vi "GetVideoInOptionsConfig.vi"(7 "HTTP_address":string, 8 "error in (no error)":errorcluster, 10 "Value":T2, 11 "Refnum in":T1) -> (0 "error out":errorcluster, 3 "headers":string)   [LabVIEW 2016]
uses:
  cgi_string.ctl
  <vilib>/httpClient/ClientHandle.ctl
  <vilib>/httpClient/LabVIEWHTTPClient.lvlib
panel:
  out "http:":string
  out "body":string
  out "Table Control":string[][](table)
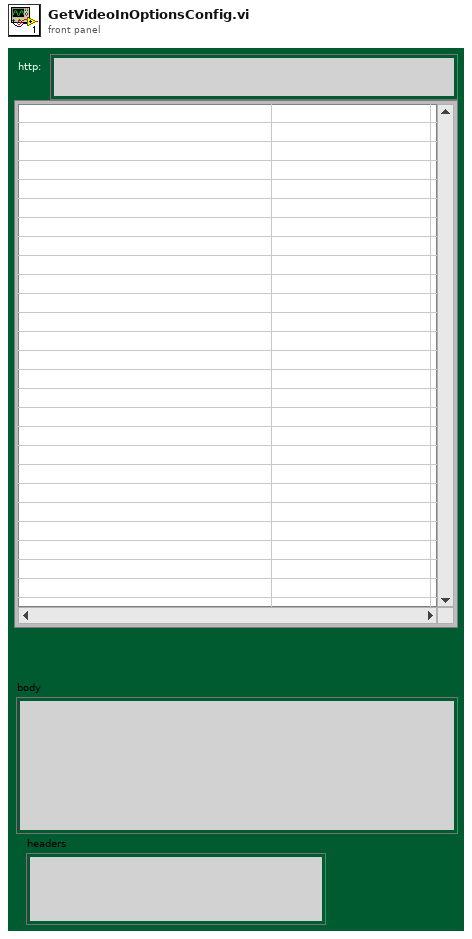
[diagram p1: front panel]
types:
  T1 = typedef "LabVIEWHTTPClient.lvlib/ClientHandle.ctl" = refnum<k1>
  T2 = typedef "cgi_string.ctl" = string
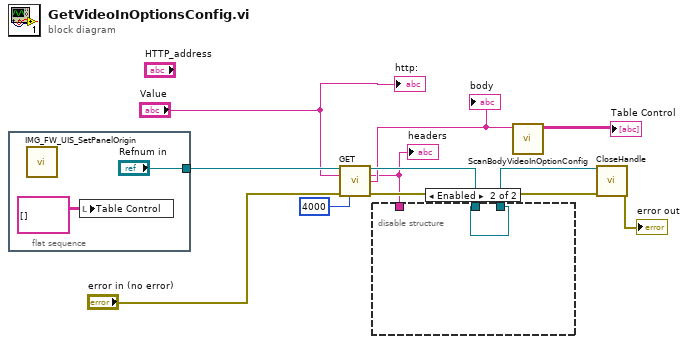
[diagram p0: block diagram]
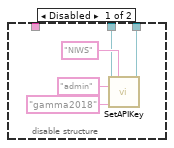
[diagram p2: hidden frame]
diagram:
  n1 = flat-sequence {
    tunnel: ["Refnum in"] -> w8
    frame #0 {
      n2 = call "IMG_FW_UIS_SetPanelOrigin.vi"() -> ()  [unwired: 11 in, 1 out]
      n3 = local write "Table Control"(string[][] [] ("Table Control")) -> ()
    }
  }
  n4 = call <vilib>:"GET.vi"("client handle"=w8, "url"="Value", "error in (no error)"="error in (no error)", "timeout (10000)"=4000) -> ("client handle out"=w7:T1, "headers"=w3:string, "body"=w5:string, "error out"=w11:errorcluster)  [unwired: 8 in]
  "body" <- w5
  "headers" <- w3
  n5 = disable-structure shown="Enabled" {
    disable-tunnel: w7 -> [w15 w19]
    disable-tunnel: [w14 w19] -> w6
    disable-tunnel: w3 -> [_ _]
    frame Disabled {
      n6 = call <vilib>:"SetAPIKey.vi"("client handle"=w15, "mode"="NIWS", "access id"="admin", "secret id"="gamma2018") -> ("client handle out"=w14:T1)  [unwired: 10 in, 1 out]
    }
    frame Enabled {
    }
  }
  n7 = call "ScanBodyVideoInOptionConfig.vi"("body"=w5) -> ("array type (2D Dbl)"=→"Table Control":string[][])  [unwired: 10 in]
  n8 = call <vilib>:"CloseHandle.vi"("client handle"=w6, "error in (no error)"=w11) -> ("error out"=→"error out":errorcluster)  [unwired: 13 in]
  "http:" <- "Value"
